vi "starburst state machine.vi"(11 "starburst in":refnum<class "starburst.lvclass">) -> ()   [LabVIEW 2015, in "starburst.lvclass"]
uses:
  starburst.lvclass
  message/communicator message.lvclass
  communicator/communicator.lvclass/communicator.ctl
  connection/connection maintainer.lvclass
  message/communicator message.lvclass/communicator message.ctl
  communicator/communicator.lvclass
  communicator/enqueue variety.ctl
  manager/new communicator message.ctl
  manager/queue manager.lvclass
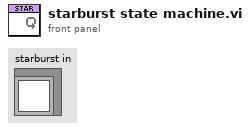
[diagram p1: front panel]
types:
  T1 = typedef "communicator.lvclass/enqueue variety.ctl" = enum16{"normal", "lossy", "priority"}
  T2 = typedef "queue manager.lvclass/new communicator message.ctl" = cluster{"ID":string, "comm":refnum<class "communicator.lvclass">}
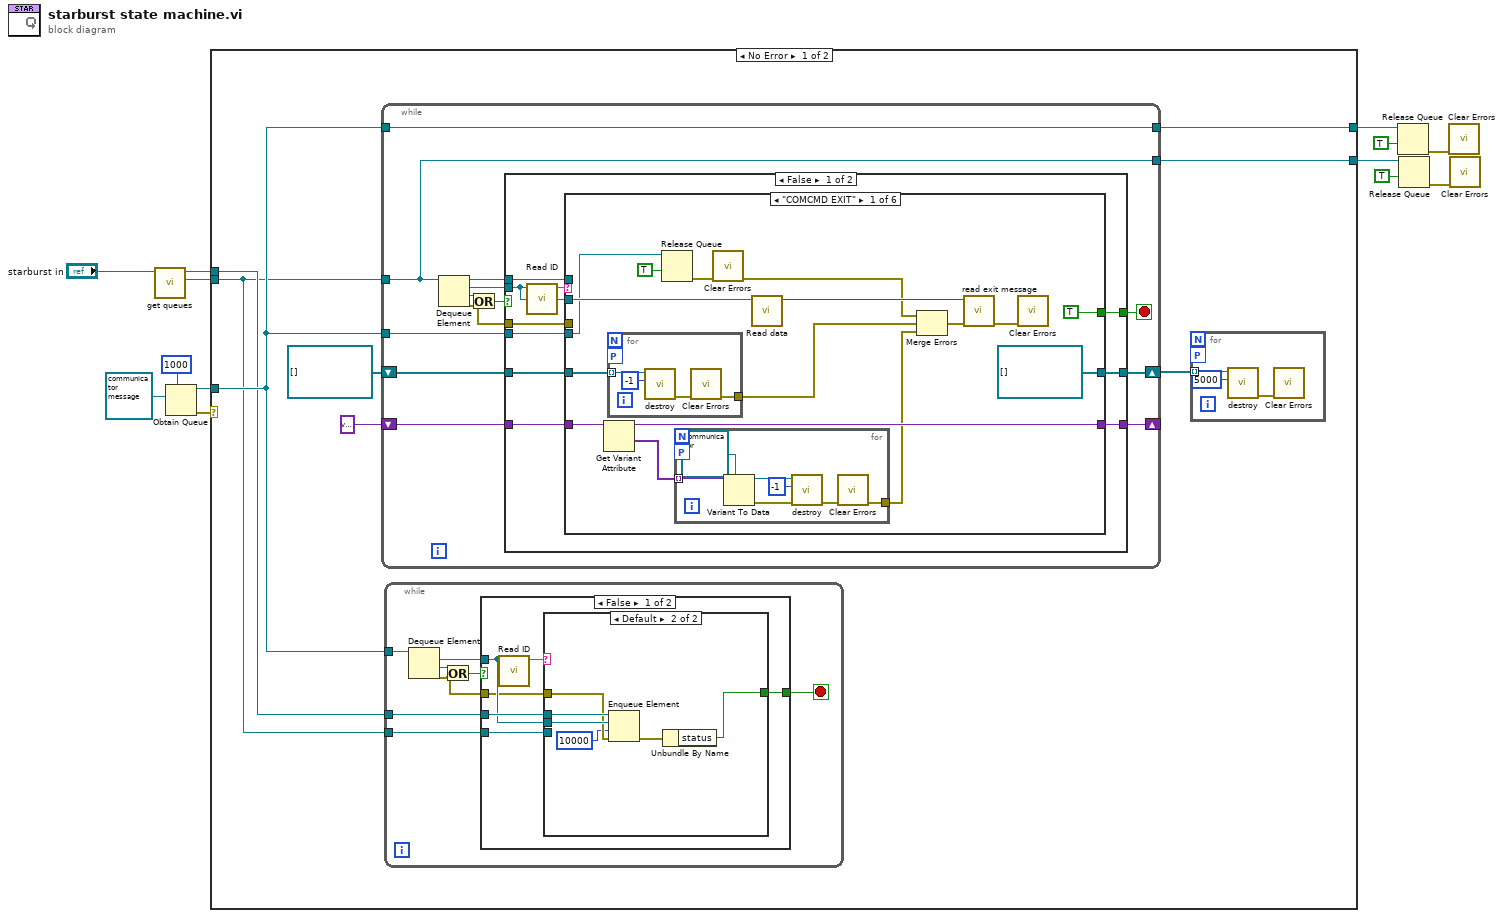
[diagram p0: block diagram]
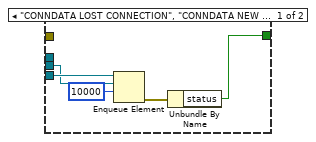
[diagram p2: hidden frame]
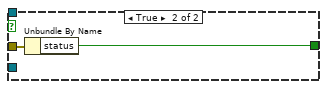
[diagram p3: hidden frame]
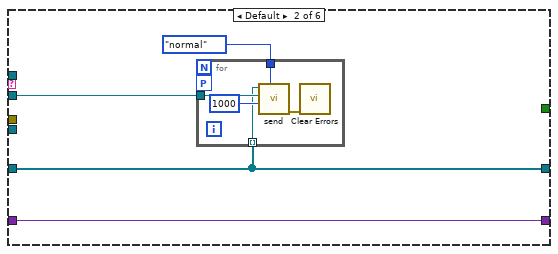
[diagram p4: hidden frame]
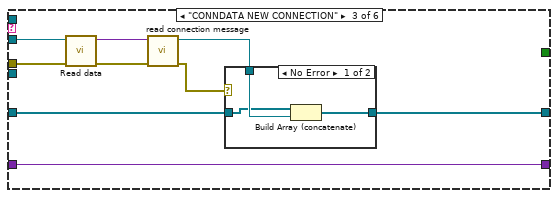
[diagram p5: hidden frame]
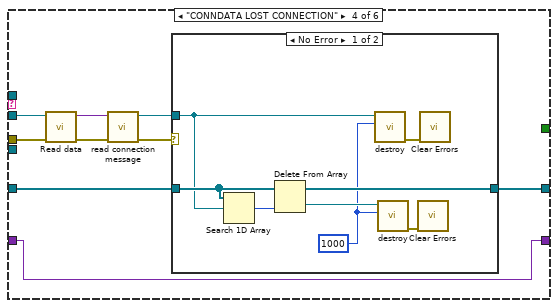
[diagram p7: hidden frame]
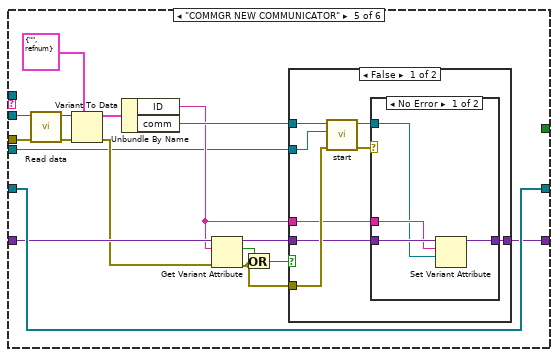
[diagram p9: hidden frame]
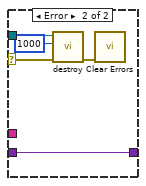
[diagram p10: hidden frame]
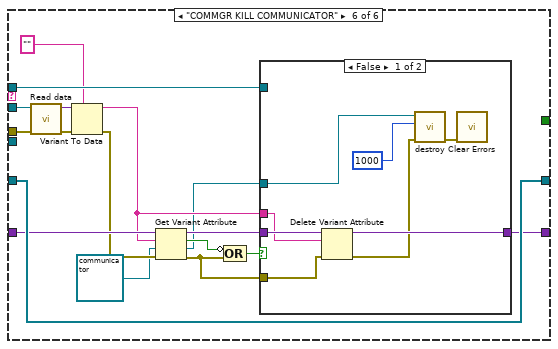
[diagram p12: hidden frame]
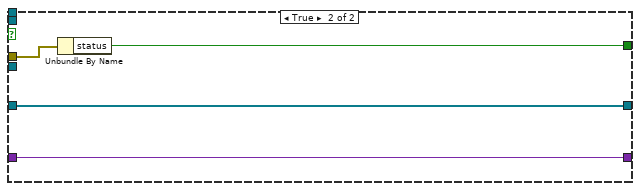
[diagram p14: hidden frame]
diagram:
  n1 = call "get queues.vi"("communicator in"="starburst in") -> ("to worker"=w12:refnum<queue>, "to parent"=w11:refnum<queue>)  [unwired: 9 in]
  n2 = Obtain Queue(max queue size (-1, unlimited)=1000, element data type=refnum<class "communicator message.lvclass"> refnum ("communicator message.lvclass")) -> (queue out=w2:refnum<queue>, error out=w5:errorcluster)  [unwired: 3 in, 1 out]
  n3 = case shown="No Error" w5 {
    tunnel: w12 -> [w14 w204]
    tunnel: w11 -> [w15 _]
    tunnel: [w21 w204] -> w10
    tunnel: w2 -> [w16 w203]
    tunnel: [w17 w203] -> w1
    frame No Error {
      n4 = while {
        tunnel: w14 -> [w58]
        tunnel: [w58] -> w21
        shift-right: [w57] -> w19
        shift-left: refnum<class "connection maintainer.lvclass">[] [] -> [w56]
        shift-right: [w54] -> _
        shift-left: variant -> [w55]
        tunnel: [w53] -> w17
        tunnel: w16 -> [w53]
        tunnel: w16 -> [w52]
        stop <- w61 stop-if-true
        n5 = Dequeue Element(queue=w58) -> (queue out=w60:refnum<queue>, element=w59:refnum<class "communicator message.lvclass">, timed out?=w64:bool, error out=w62:errorcluster)  [unwired: 2 in]
        n6 = Or(x=w64, y=w62) -> (x .or. y?=w63:bool)
        n7 = case shown="False" w63 {
          tunnel: w62 -> [w71 w202]
          tunnel: [w73 w201] -> w61
          tunnel: w60 -> [w66 _]
          tunnel: w59 -> [w72 _]
          tunnel: [w70 w200] -> w57
          tunnel: w56 -> [w69 w200]
          tunnel: w55 -> [w68 w199]
          tunnel: [w67 w199] -> w54
          tunnel: w52 -> [w65 _]
          frame False {
            n8 = call "Read ID.vi"("communicator message in"=w72) -> ("ID"=w74:string)  [unwired: 10 in]
            n9 = case shown="\"COMCMD EXIT\"" w74 {
              tunnel: [TRUE _ _ _ _ _] -> w73
              tunnel: w72 -> [w89 w102 w118 w129 w154 w188]
              tunnel: w71 -> [_ _ w117 w130 w152 w186]
              tunnel: [refnum<class "connection maintainer.lvclass">[] [] w105 w115 w127 w155 w189] -> w70
              tunnel: w69 -> [w87 w105 w114 w126 w155 w189]
              tunnel: w68 -> [w84 w104 w112 w124 w149 w185]
              tunnel: [w83 w104 w112 w124 w144 w180] -> w67
              tunnel: w66 -> [_ _ _ _ _ w178]
              tunnel: w65 -> [w76 _ _ _ w140 _]
              frame "COMCMD EXIT" {
                n10 = Get Variant Attribute(Variant=w84) -> (duplicate Variant=w83:variant, values=w82:variant[])  [unwired: 3 in, 2 out]
                n11 = for {
                  tunnel: w87 -> [w100] mode=indexing
                  workers-P: _ -> [_]
                  tunnel: [w98] -> w85
                  n12 = call-dynamic "destroy.vi"("timeout in ms (-1)"=-1, "communicator in"=w100) -> ("error out"=w101:errorcluster)  [unwired: 9 in]
                  n13 = call <vilib>:"Clear Errors.vi"("error in (no error)"=w101) -> ("error out"=w98:errorcluster)  [unwired: 5 in, 1 out]
                }
                n14 = Release Queue(queue=w76, force destroy? (F)=TRUE) -> (error out=w78:errorcluster)  [unwired: 1 in, 2 out]
                n15 = for {
                  tunnel: w82 -> [w96] mode=indexing
                  workers-P: _ -> [_]
                  tunnel: [w94] -> w80
                  n16 = Variant To Data(type=refnum<class "communicator.lvclass"> refnum ("communicator.lvclass"), Variant=w96) -> (data=w91:refnum<class "communicator.lvclass">, error out=w93:errorcluster)  [unwired: 1 in]
                  n17 = call-dynamic "destroy.vi"("error in"=w93, "timeout in ms (-1)"=-1, "communicator in"=w91) -> ("error out"=w97:errorcluster)  [unwired: 8 in]
                  n18 = call <vilib>:"Clear Errors.vi"("error in (no error)"=w97) -> ("error out"=w94:errorcluster)  [unwired: 5 in, 1 out]
                }
                n19 = call <vilib>:"Clear Errors.vi"("error in (no error)"=w78) -> ("error out"=w75:errorcluster)  [unwired: 5 in, 1 out]
                n20 = call "Read data.vi"("communicator message in"=w89) -> ("data"=w79:variant)  [unwired: 10 in]
                n21 = Merge Errors(w75, w85, w80) -> (w81:errorcluster)
                n22 = call "read exit message.vi"("error in"=w81, "data"=w79) -> ("error out"=w88:errorcluster)  [unwired: 9 in]
                n23 = call <vilib>:"Clear Errors.vi"("error in (no error)"=w88) -> ()  [unwired: 5 in, 2 out]
              }
              frame Default {
                n24 = for {
                  workers-P: _ -> [_]
                  tunnel: w102 -> [w110]
                  tunnel: enqueue_variety."normal" ("enqueue setting") -> [w109]
                  tunnel: w105 -> [w107] mode=indexing
                  n25 = call "send.vi"("enqueue setting"=w109, "timeout in ms (-1)"=1000, "element"=w110, "communicator in"=w107) -> ("error out"=w106:errorcluster)  [unwired: 7 in]
                  n26 = call <vilib>:"Clear Errors.vi"("error in (no error)"=w106) -> ()  [unwired: 5 in, 2 out]
                }
              }
              frame "CONNDATA NEW CONNECTION" {
                n27 = call "Read data.vi"("communicator message in"=w118) -> ("data"=w111:variant)  [unwired: 10 in]
                n28 = call "read connection message.vi"("error in"=w117, "data"=w111) -> ("error out"=w113:errorcluster, "conn"=w116:refnum<class "connection maintainer.lvclass">)  [unwired: 8 in]
                n29 = case shown="No Error" w113 {
                  tunnel: w116 -> [w121 _]
                  tunnel: [w120 w122] -> w115
                  tunnel: w114 -> [w119 w122]
                  frame No Error {
                    n30 = Build Array (concatenate)(w119, w121) -> (w120:refnum<class "connection maintainer.lvclass">[])
                  }
                  frame Error {
                  }
                }
              }
              frame "CONNDATA LOST CONNECTION" {
                n31 = call "Read data.vi"("communicator message in"=w129) -> ("data"=w123:variant)  [unwired: 10 in]
                n32 = call "read connection message.vi"("error in"=w130, "data"=w123) -> ("error out"=w128:errorcluster, "conn"=w125:refnum<class "connection maintainer.lvclass">)  [unwired: 8 in]
                n33 = case shown="No Error" w128 {
                  tunnel: [w136 w139] -> w127
                  tunnel: w126 -> [w137 w139]
                  tunnel: w125 -> [w134 _]
                  frame No Error {
                    w133 = 1000 ("timeout in ms (-1)")
                    n34 = Search 1D Array(1D array=w137, element=w134) -> (index of element=w138:i32)  [unwired: 1 in]
                    n35 = Delete From Array(array=w137, index=w138) -> (deleted portion=w135:refnum<class "connection maintainer.lvclass">, array with subset deleted=w136:refnum<class "connection maintainer.lvclass">[])  [unwired: 1 in]
                    n36 = call-dynamic "destroy.vi"("timeout in ms (-1)"=w133, "communicator in"=w134) -> ("error out"=w132:errorcluster)  [unwired: 9 in]
                    n37 = call-dynamic "destroy.vi"("timeout in ms (-1)"=w133, "communicator in"=w135) -> ("error out"=w131:errorcluster)  [unwired: 9 in]
                    n38 = call <vilib>:"Clear Errors.vi"("error in (no error)"=w131) -> ()  [unwired: 5 in, 2 out]
                    n39 = call <vilib>:"Clear Errors.vi"("error in (no error)"=w132) -> ()  [unwired: 5 in, 2 out]
                  }
                  frame Error {
                  }
                }
              }
              frame "COMMGR NEW COMMUNICATOR" {
                n40 = call "Read data.vi"("communicator message in"=w154) -> ("data"=w153:variant)  [unwired: 10 in]
                n41 = Variant To Data(error in=w152, type=T2 {"ID"="", "comm"=refnum} ("new comm message"), Variant=w153) -> (data=w150:T2, error out=w148:errorcluster)
                n42 = Unbundle By Name(w150) -> ("ID"=w141:string, "comm"=w142:refnum<class "communicator.lvclass">)
                n43 = Get Variant Attribute(Variant=w149, name=w141, error in=w148) -> (duplicate Variant=w145:variant, found=w147:bool, error out=w143:errorcluster)  [unwired: 1 in, 1 out]
                n44 = Or(x=w147, y=w143) -> (x .or. y?=w146:bool)
                n45 = case shown="False" w146 {
                  tunnel: w145 -> [w161 w173]
                  tunnel: [w160 w173] -> w144
                  tunnel: w143 -> [w162 _]
                  tunnel: w142 -> [w163 _]
                  tunnel: w141 -> [w159 _]
                  tunnel: w140 -> [w156 _]
                  frame False {
                    n46 = call-dynamic "start.vi"("error in"=w162, "queue to parent"=w156, "communicator in"=w163) -> ("error out"=w157:errorcluster, "communicator out"=w158:refnum<class "communicator.lvclass">)  [unwired: 7 in]
                    n47 = case shown="No Error" w157 {
                      selector: w157 -> [_ w170]
                      tunnel: w161 -> [w167 w172]
                      tunnel: [w166 w172] -> w160
                      tunnel: w159 -> [w165 _]
                      tunnel: w158 -> [w164 w171]
                      frame No Error {
                        n48 = Set Variant Attribute(Variant=w167, name=w165, value=w164) -> (Variant out=w166:variant)  [unwired: 1 in, 2 out]
                      }
                      frame Error {
                        n49 = call-dynamic "destroy.vi"("error in"=w170, "timeout in ms (-1)"=1000, "communicator in"=w171) -> ("error out"=w168:errorcluster)  [unwired: 8 in]
                        n50 = call <vilib>:"Clear Errors.vi"("error in (no error)"=w168) -> ()  [unwired: 5 in, 2 out]
                      }
                    }
                  }
                  frame True {
                    # "error or exists"
                  }
                }
              }
              frame "COMMGR KILL COMMUNICATOR" {
                n51 = call "Read data.vi"("communicator message in"=w188) -> ("data"=w187:variant)  [unwired: 10 in]
                n52 = Variant To Data(error in=w186, type="", Variant=w187) -> (data=w176:string, error out=w184:errorcluster)
                n53 = Get Variant Attribute(Variant=w185, name=w176, default value (empty Variant)=refnum<class "communicator.lvclass"> refnum ("communicator out"), error in=w184) -> (duplicate Variant=w181:variant, found=w183:bool, value=w174:refnum<class "communicator.lvclass">, error out=w179:errorcluster)
                n54 = Compound Arithmetic op=OR(invert w183, w179) -> (w182:bool)
                n55 = case shown="False" w182 {
                  tunnel: w181 -> [w197 w198]
                  tunnel: [w193 w198] -> w180
                  tunnel: w179 -> [w191 _]
                  tunnel: w176 -> [w192 _]
                  tunnel: w178 -> [_ _]
                  tunnel: w174 -> [w194 _]
                  frame False {
                    n56 = Delete Variant Attribute(4:w191, 6:w192, 7:w197) -> (0:w190:errorcluster, 3:w193:variant)  [unwired: 1 out]
                    n57 = call-dynamic "destroy.vi"("error in"=w190, "timeout in ms (-1)"=1000, "communicator in"=w194) -> ("error out"=w195:errorcluster)  [unwired: 8 in]
                    n58 = call <vilib>:"Clear Errors.vi"("error in (no error)"=w195) -> ()  [unwired: 5 in, 2 out]
                  }
                  frame True {
                    # "error or not exists"
                  }
                }
              }
            }
          }
          frame True {
            n59 = Unbundle By Name(w202) -> ("status"=w201:bool)
          }
        }
      }
      n60 = while {
        tunnel: w16 -> [w28]
        tunnel: w15 -> [w23]
        tunnel: w14 -> [w22]
        stop <- w25 stop-if-true
        n61 = Dequeue Element(queue=w28) -> (element=w24:refnum<class "communicator message.lvclass">, timed out?=w29:bool, error out=w26:errorcluster)  [unwired: 2 in, 1 out]
        n62 = Or(x=w29, y=w26) -> (x .or. y?=w27:bool)
        n63 = case shown="False" w27 {
          tunnel: w26 -> [w32 w48]
          tunnel: [w31 w47] -> w25
          tunnel: w24 -> [w33 _]
          tunnel: w23 -> [w34 _]
          tunnel: w22 -> [w30 _]
          frame False {
            n64 = call "Read ID.vi"("communicator message in"=w33) -> ("ID"=w35:string)  [unwired: 10 in]
            n65 = case shown="Default" w35 {
              tunnel: w34 -> [_ w46]
              tunnel: w33 -> [w38 w45]
              tunnel: w32 -> [_ w44]
              tunnel: [w37 w42] -> w31
              tunnel: w30 -> [w39 _]
              frame "CONNDATA LOST CONNECTION", "CONNDATA NEW CONNECTION" {
                n66 = Enqueue Element(queue=w39, element=w38, timeout in ms (-1)=10000) -> (error out=w40:errorcluster)  [unwired: 1 in, 2 out]
                n67 = Unbundle By Name(w40) -> ("status"=w37:bool)
              }
              frame Default {
                n68 = Enqueue Element(queue=w46, element=w45, timeout in ms (-1)=10000, error in (no error)=w44) -> (error out=w43:errorcluster)  [unwired: 2 out]
                n69 = Unbundle By Name(w43) -> ("status"=w42:bool)
              }
            }
          }
          frame True {
            n70 = Unbundle By Name(w48) -> ("status"=w47:bool)
          }
        }
      }
      n71 = for {
        tunnel: w19 -> [w50] mode=indexing
        workers-P: _ -> [_]
        n72 = call-dynamic "destroy.vi"("timeout in ms (-1)"=5000, "communicator in"=w50) -> ("error out"=w51:errorcluster)  [unwired: 9 in]
        n73 = call <vilib>:"Clear Errors.vi"("error in (no error)"=w51) -> ()  [unwired: 5 in, 2 out]
      }
    }
    frame Error {
    }
  }
  n74 = Release Queue(queue=w1, force destroy? (F)=TRUE) -> (error out=w4:errorcluster)  [unwired: 1 in, 2 out]
  n75 = Release Queue(queue=w10, force destroy? (F)=TRUE) -> (error out=w8:errorcluster)  [unwired: 1 in, 2 out]
  n76 = call <vilib>:"Clear Errors.vi"("error in (no error)"=w4) -> ()  [unwired: 5 in, 2 out]
  n77 = call <vilib>:"Clear Errors.vi"("error in (no error)"=w8) -> ()  [unwired: 5 in, 2 out]
